vi "Remove Duplicates from Numeric DBL 1D Array.vi"(7 "Tolerance (1E-9)":dbl=1e-09, 8 "error in (no error)":errorcluster, 9 "Array In":dbl[](array[numeric])) -> (0 "error out":errorcluster, 1 "Sorted Array with Duplicates Removed":dbl[](array[numeric]))   [LabVIEW 2010]
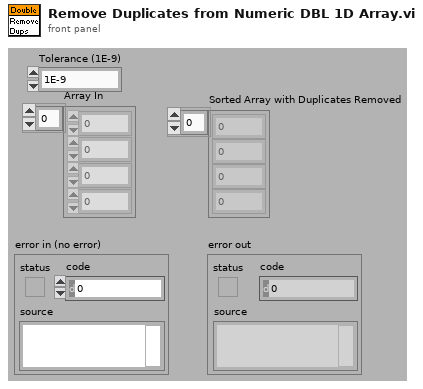
[diagram p1: front panel]
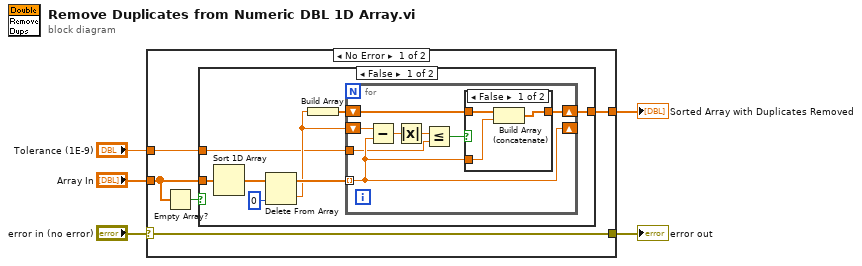
[diagram p0: block diagram]
diagram:
  n1 = case shown="No Error" "error in (no error)" {
    selector: "error in (no error)" -> [w10 w32]
    tunnel: [w10 w32] -> w4
    tunnel: "Array In" -> [w7 _]
    tunnel: [w9 _] -> w2
    tunnel: "Tolerance (1E-9)" -> [w8 _]
    frame No Error {
      n2 = Empty Array?(array=w7) -> (empty?=w6:bool)
      n3 = case shown="False" w6 {
        tunnel: [w18 w31] -> w9
        tunnel: w8 -> [w12 _]
        tunnel: w7 -> [w11 w31]
        frame False {
          n4 = Sort 1D Array(array=w11) -> (sorted array=w17:dbl[])
          n5 = Delete From Array(array=w17, index=0) -> (deleted portion=w14:dbl, array with subset deleted=w16:dbl[])  [unwired: 1 in]
          n6 = Build Array(w14) -> (w13:dbl[])
          n7 = for {
            tunnel: w16 -> [w23] mode=indexing
            shift-right: [w25] -> w18
            shift-left: w13 -> [w26]
            shift-right: [w23] -> _
            shift-left: w14 -> [w24]
            tunnel: w12 -> [w20]
            n8 = Subtract(x=w24, y=w23) -> (x-y=w22:dbl)
            n9 = Absolute Value(x=w22) -> (abs(x)=w21:dbl)
            n10 = Less Or Equal?(x=w21, y=w20) -> (x <= y?=w19:bool)
            n11 = case shown="False" w19 {
              tunnel: w26 -> [w29 w30]
              tunnel: [w28 w30] -> w25
              tunnel: w23 -> [w27 _]
              frame False {
                n12 = Build Array (concatenate)(w29, w27) -> (w28:dbl[])
              }
              frame True {
              }
            }
          }
        }
        frame True {
        }
      }
    }
    frame Error {
    }
  }
  "Sorted Array with Duplicates Removed" <- w2
  "error out" <- w4
